vi "Reset.vi"(7 "Direction (all)":T2(ring), 8 "error in (no error)":errorcluster, 11 "PongBall in":refnum<class "PongBall.lvclass">) -> (0 "error out":errorcluster, 3 "PongBall out":refnum<class "PongBall.lvclass">)   [LabVIEW 2019, in "RT_Game.lvlib" / "PongBall.lvclass"]
uses:
  PongBall.lvclass
  C:/Users/FreshBob/Dropbox/VIs/myRIO_GameConsole/RT/RT_Game/GameObject/GameObject.lvclass
  Velocity.ctl
  PongBall.lvclass/PongBall.ctl
  GameObject/GameObject.lvclass/GameObject.ctl
  GameObject/Read MaxSpeed.vi
  GameObject/Read MinSpeed.vi
  GameObject/Write last_position.vi
  GameObject/Read MaxSpeedX.vi
  GameObject/Read MinSpeedX.vi
  GameObject/Write Velocity.vi
  GameObject/GameObject.lvclass
  RT_Game.lvlib
panel:
  in  "Velocity":T1
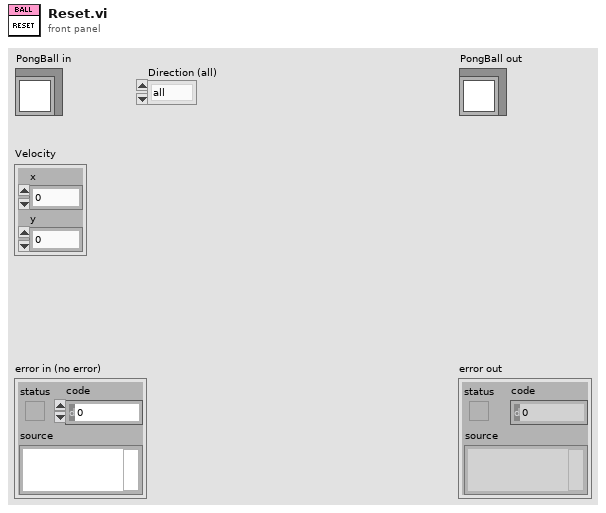
[diagram p1: front panel]
types:
  T1 = typedef "RT_Game.lvlib/Velocity.ctl" = cluster{"x":dbl, "y":dbl}
  T2 = enum16{"all", "up", "down", "left", "right", "leftup", "rightup", "leftdown", "rightdown"}
  T3 = typedef "RT_Game.lvlib/Engine.lvclass/Coordinate.ctl" = cluster{"x":dbl, "y":dbl}
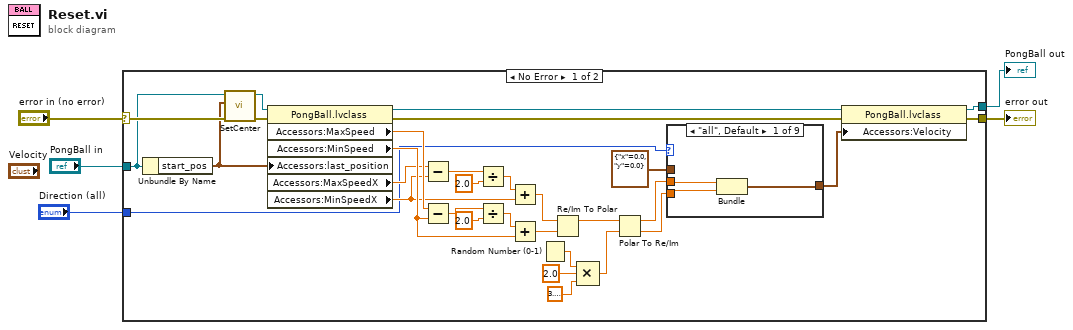
[diagram p0: block diagram]
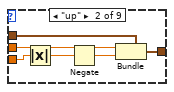
[diagram p2: hidden frame]
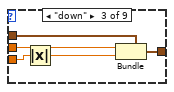
[diagram p3: hidden frame]
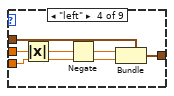
[diagram p4: hidden frame]
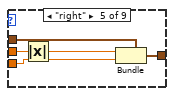
[diagram p5: hidden frame]
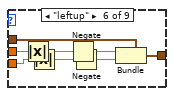
[diagram p6: hidden frame]
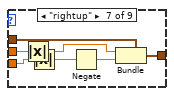
[diagram p7: hidden frame]
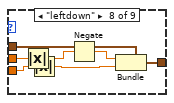
[diagram p8: hidden frame]
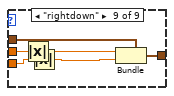
[diagram p9: hidden frame]
diagram:
  n1 = case shown="No Error" "error in (no error)" {
    selector: "error in (no error)" -> [w36 w91]
    tunnel: [w25 w91] -> w4
    tunnel: [w24 w90] -> w2
    tunnel: "PongBall in" -> [w17 w90]
    tunnel: "Direction (all)" -> [w6 _]
    frame No Error {
      n2 = Unbundle By Name(w17) -> ("start_pos"=w16:T3)
      n3 = call "SetCenter.vi"("error in (no error)"=w36, "center_position"=w16, "GameObject in"=w17) -> ("error out"=w35:errorcluster, "GameObject out"=w21:refnum<class "PongBall.lvclass">)  [unwired: 7 in]
      n4 = property class="PongBall.lvclass"(reference=w21, error in=w35, "Accessors:last_position"=w16) -> (reference out=w18:refnum<class "PongBall.lvclass">, error out=w22:errorcluster, "Accessors:MaxSpeed"=w20:dbl, "Accessors:MinSpeed"=w19:dbl, "Accessors:MaxSpeedX"=w9:dbl, "Accessors:MinSpeedX"=w10:dbl)
      n5 = Subtract(x=w9, y=w10) -> (x-y=w12:dbl)
      n6 = Subtract(x=w20, y=w19) -> (x-y=w11:dbl)
      n7 = Divide(x=w12, y=2.0) -> (x/y=w14:dbl)
      n8 = Divide(x=w11, y=2.0) -> (x/y=w33:dbl)
      n9 = Add(x=w14, y=w10) -> (x+y=w8:dbl)
      n10 = Add(x=w33, y=w19) -> (x+y=w15:dbl)
      n11 = Random Number (0-1)() -> (number: 0 to 1=w31:dbl)
      n12 = Re/Im To Polar(2:w15, 3:w8) -> (1:w7:dbl)  [unwired: 1 out]
      n13 = Compound Arithmetic op=MULTIPLY(w31, 2.0 ("y"), 3.141592653589793) -> (w28:dbl)
      n14 = Polar To Re/Im(2:w28, 3:w7) -> (0:w26:dbl, 1:w27:dbl)
      n15 = case shown="\"all\", Default" w6 {
        tunnel: T1 {"x"=0.0, "y"=0.0} ("Velocity") -> [_ w45 w50 w56 w61 w69 w76 w83 w89]
        tunnel: w27 -> [w39 w44 w49 w55 w60 w68 w75 w82 w88]
        tunnel: w26 -> [w38 w43 w48 w53 w58 w66 w73 w80 w86]
        tunnel: [w37 w42 w47 w54 w59 w67 w74 w81 w87] -> w23
        frame "all", Default {
          n16 = Bundle(w39, w38) -> (w37:cluster{dbl, dbl})  [unwired: 1 in]
        }
        frame "up" {
          n17 = Absolute Value(x=w43) -> (abs(x)=w41:dbl)
          n18 = Negate(x=w41) -> (-x=w40:dbl)
          n19 = Bundle(cluster=w45, "x"=w44, "y"=w40) -> (w42:T1)
        }
        frame "down" {
          n20 = Absolute Value(x=w48) -> (abs(x)=w46:dbl)
          n21 = Bundle(cluster=w50, "x"=w49, "y"=w46) -> (w47:T1)
        }
        frame "left" {
          n22 = Absolute Value(x=w55) -> (abs(x)=w52:dbl)
          n23 = Negate(x=w52) -> (-x=w51:dbl)
          n24 = Bundle(cluster=w56, "x"=w51, "y"=w53) -> (w54:T1)
        }
        frame "right" {
          n25 = Absolute Value(x=w60) -> (abs(x)=w57:dbl)
          n26 = Bundle(cluster=w61, "x"=w57, "y"=w58) -> (w59:T1)
        }
        frame "leftup" {
          n27 = Absolute Value(x=w68) -> (abs(x)=w65:dbl)
          n28 = Absolute Value(x=w66) -> (abs(x)=w64:dbl)
          n29 = Negate(x=w65) -> (-x=w63:dbl)
          n30 = Negate(x=w64) -> (-x=w62:dbl)
          n31 = Bundle(cluster=w69, "x"=w63, "y"=w62) -> (w67:T1)
        }
        frame "rightup" {
          n32 = Absolute Value(x=w75) -> (abs(x)=w72:dbl)
          n33 = Absolute Value(x=w73) -> (abs(x)=w71:dbl)
          n34 = Negate(x=w71) -> (-x=w70:dbl)
          n35 = Bundle(cluster=w76, "x"=w72, "y"=w70) -> (w74:T1)
        }
        frame "leftdown" {
          n36 = Absolute Value(x=w82) -> (abs(x)=w79:dbl)
          n37 = Absolute Value(x=w80) -> (abs(x)=w77:dbl)
          n38 = Negate(x=w79) -> (-x=w78:dbl)
          n39 = Bundle(cluster=w83, "x"=w78, "y"=w77) -> (w81:T1)
        }
        frame "rightdown" {
          n40 = Absolute Value(x=w88) -> (abs(x)=w84:dbl)
          n41 = Absolute Value(x=w86) -> (abs(x)=w85:dbl)
          n42 = Bundle(cluster=w89, "x"=w84, "y"=w85) -> (w87:T1)
        }
      }
      n43 = property class="PongBall.lvclass"(reference=w18, error in=w22, "Accessors:Velocity"=w23) -> (reference out=w24:refnum<class "PongBall.lvclass">, error out=w25:errorcluster)
    }
    frame Error {
    }
  }
  "error out" <- w4
  "PongBall out" <- w2
